vi "Main.vi"() -> ()   [LabVIEW 2014]
uses:
  Controls/FHandlerClusterTypedef.ctl
  Controls/FHandlerEnumTypedef.ctl
  Controls/CMWQCluster.ctl
  Controls/CMWQEnum.ctl
  Controls/CommentLogClusterTypedef.ctl
  Controls/CommentLogEnumTypedef.ctl
  <vilib>/Utility/sysdir.llb/System Directory Type.ctl
  Files/config/TableReference.ctl
  <vilib>/Utility/miscctls.llb/LVRowAndColumnTypeDef.ctl
  Controls/FGVisfileopen.ctl
  Controls/DataPack.ctl
  Controls/HeaderParameters.ctl
  Controls/MasterClusterTypedef.ctl
  Controls/MasterEnumTypedef.ctl
  Controls/ConfigFileWrite.ctl
  Controls/AddCommentParameters.ctl
panel:
  in  "PrintButton":bool
  out "Values going into graph":waveform(dbl)[](array[waveform])
  in  "Stop button":bool
  out "Error Out":errorcluster
  in  "Error In":errorcluster
  in  "Tab Control":T1(tab)
  out "Process GIF":bool
  in  "StartAcquisition":bool
  in  "StopAcq":bool
  in  "Clear-table":bool
  in  "Load Table from:":path=path "C:/LabVIEW Projects/coldex/COLDEX_LV_CG/trunk/Files/config/20150803_163022_configtable1.xlsx"
  in  "Table":i32(listbox)
  in  "LoadConfig":bool
  in  "ExportConfig":bool
  in  "File Path":path=path "C:/LabVIEW Projects/coldex/COLDEX_LV_CG/trunk/Documentation"
  in  "Comments:":string
  in  "Comment":bool
  in  "Clear Graph":bool
  out "Display Table":string[][](table)
  out "Output Waveforms":waveform(dbl)[](graph)
  # "EXPERIMENTAL DATA"
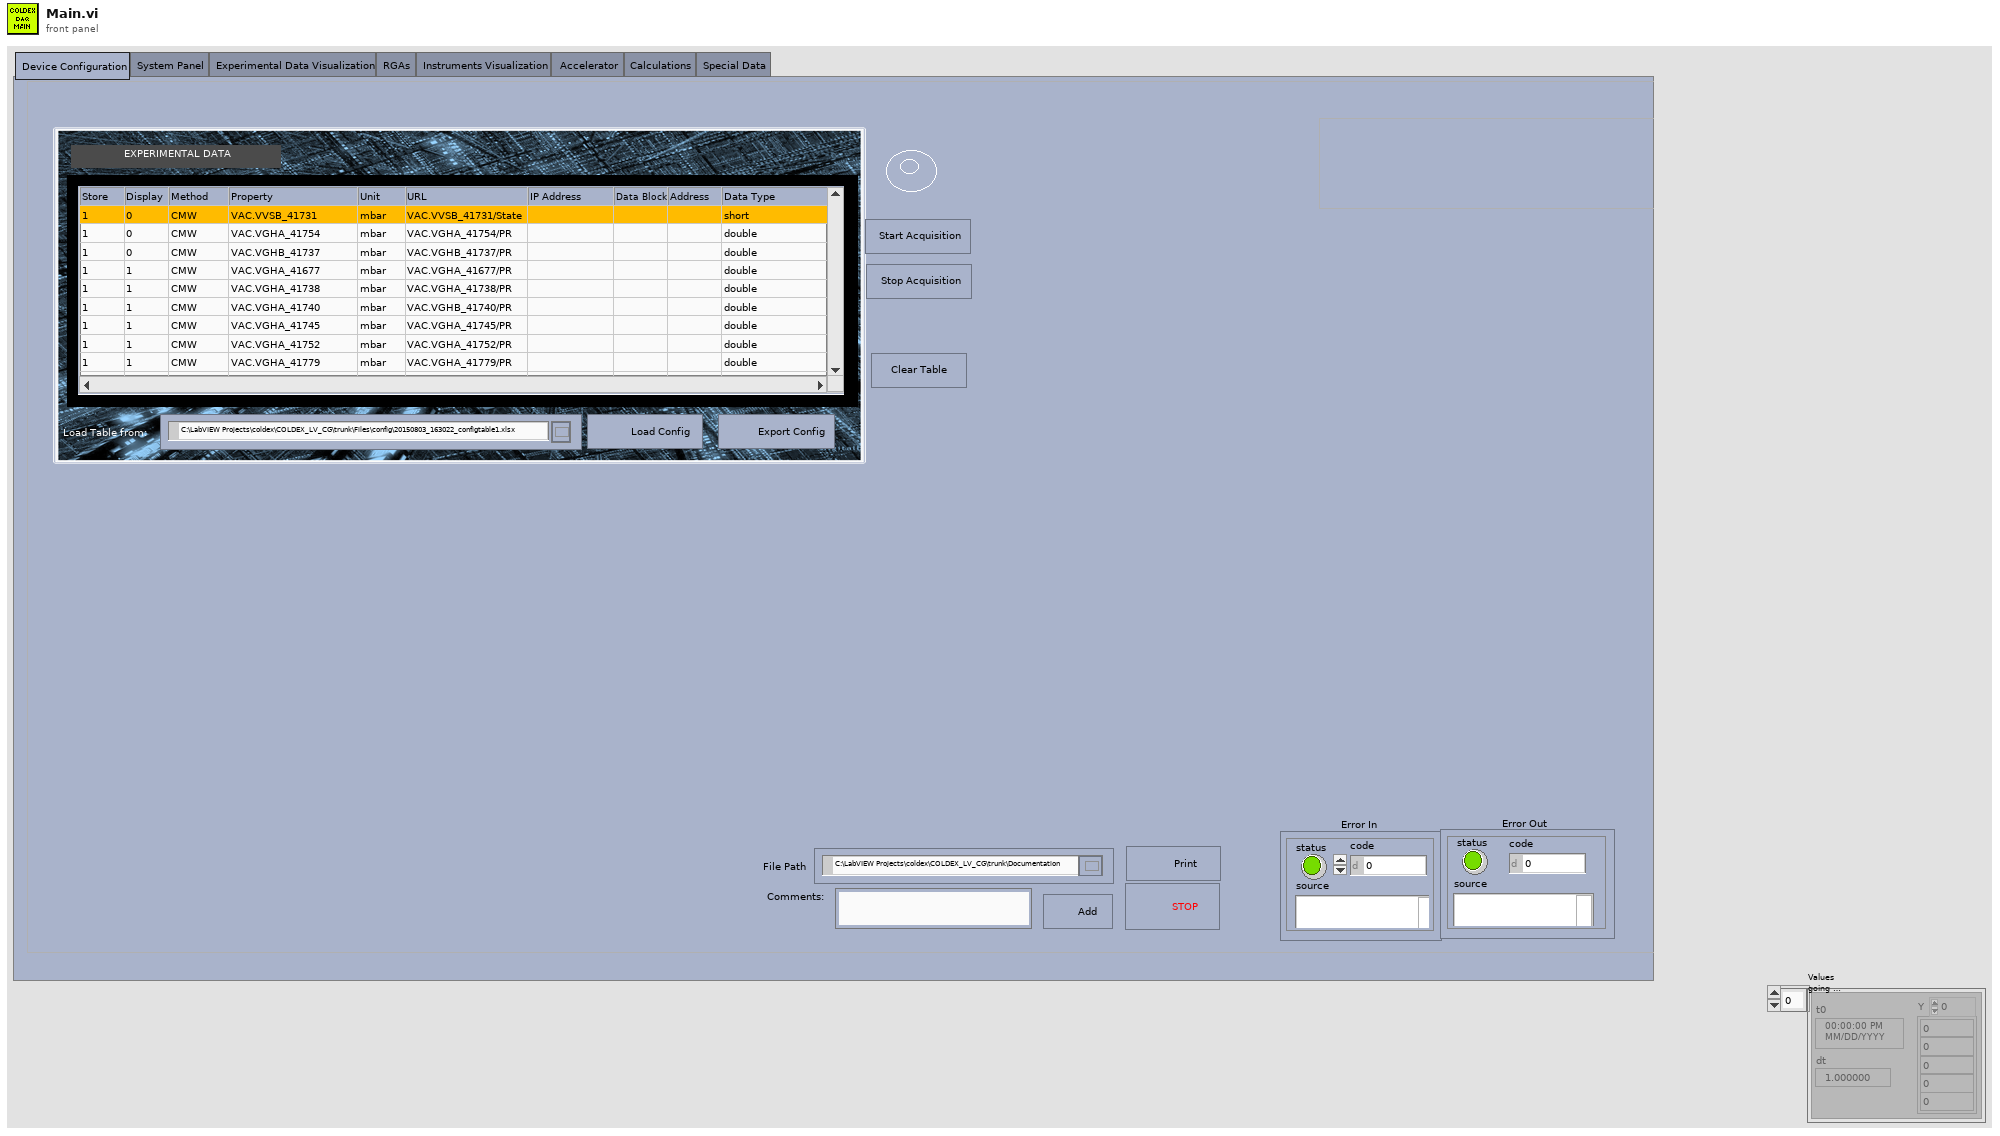
[diagram p1: front panel]
types:
  T1 = enum32{"Device Configuration", "System Panel", "Experimental Data Visualization", "RGAs", "Instruments Visualization", "Accelerator ", "Calculations", "Special Data"}
  T2 = typedef "FGVisfileopen.ctl" = enum16{"Read", "Write"}
  T3 = typedef "HeaderParameters.ctl" = cluster{"Property":string[], "Unit":string[], "Log Path":path}
  T4 = typedef "FHandlerClusterTypedef.ctl" = cluster{"File Variant":variant, "FileHandler Enum":T5}
  T5 = typedef "FHandlerEnumTypedef.ctl" = enum16{"InitLog", "CommentLog", "WriteExperimental", "WriteRGA", "WriteAccelerator", "WriteInstrument", "ClearLog", "ReadConfig", "WriteConfig", "ExitFH"}
  T6 = typedef "MasterClusterTypedef.ctl" = cluster{"DisplayVariant":variant, "DisplayEnum":T7}
  T7 = typedef "MasterEnumTypedef.ctl" = enum16{"Idle", "Initialize", "StartAcquisition", "StoreAcquisition", "PrintScreen", "AddComment", "ClearTable", "DisplayTable", "DisplayWaveforms", "ExportConfig", "LoadConfig", "Exit"}
  T8 = typedef "ConfigFileWrite.ctl" = cluster{"Headers":string[], "TableContent":string[][], "PathConfig":path}
  T9 = typedef "CommentLogClusterTypedef.ctl" = cluster{"variant":variant, "enum":T10}
  T10 = typedef "CommentLogEnumTypedef.ctl" = enum16{"AddComment", "Exit"}
  T11 = typedef "AddCommentParameters.ctl" = cluster{"PathConfig":path, "Comment":string}
  T12 = typedef "CMWQCluster.ctl" = cluster{"Variant":variant, "Enum":T13}
  T13 = typedef "CMWQEnum.ctl" = enum16{"Initialise", "Acquire", "Stop"}
  T14 = typedef "System Directory Type.ctl" = i32
  T15 = typedef "TableReference.ctl" = cluster{"Table Reference":refnum<vi>, "Cell Position":T16}
  T16 = typedef "LVRowAndColumnTypeDef.ctl" = cluster{"Row":i32, "Column":i32}
  T17 = typedef "LVPoint32TypeDef.ctl" = cluster{"Horizontal":i32, "Vertical":i32}
  T18 = cluster{"Start Row":i32, "Start Column":i32, "End Row":i32, "End Column":i32}
  T19 = typedef "DataPack.ctl" = cluster{"DataPack Array":cluster{"Method":string, "PropertyName":string, "Value":string, "Display?":string, "Unit":string}[], "current time":timestamp}
  T20 = cluster{"Method":string, "PropertyName":string, "Value":string, "Display?":string, "Unit":string}[]
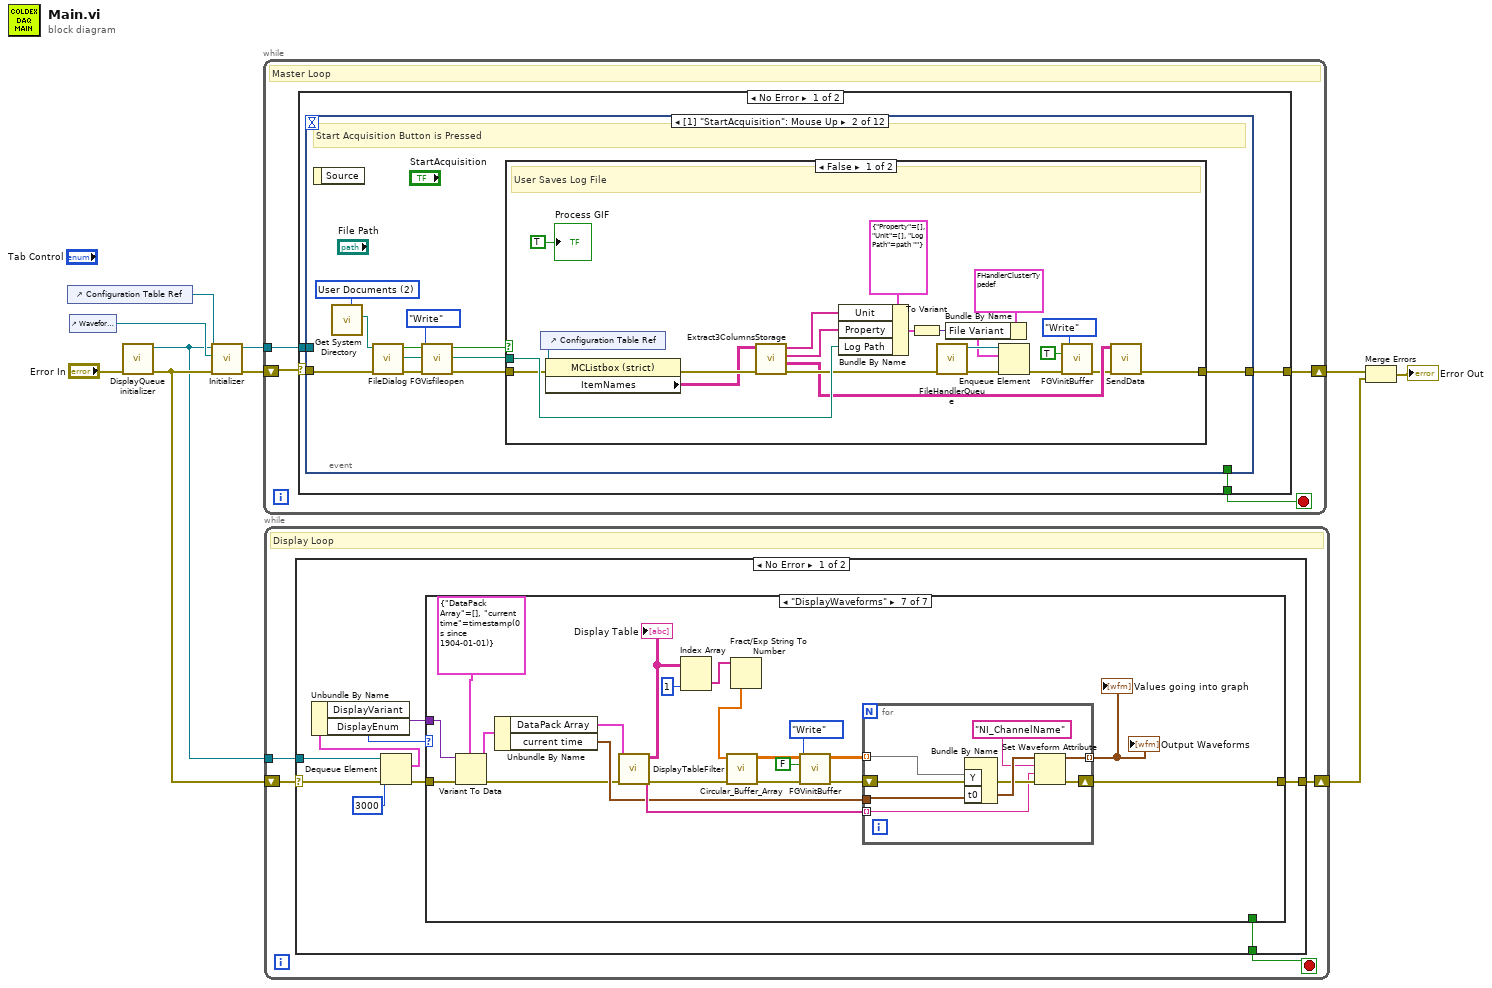
[diagram p0: block diagram]
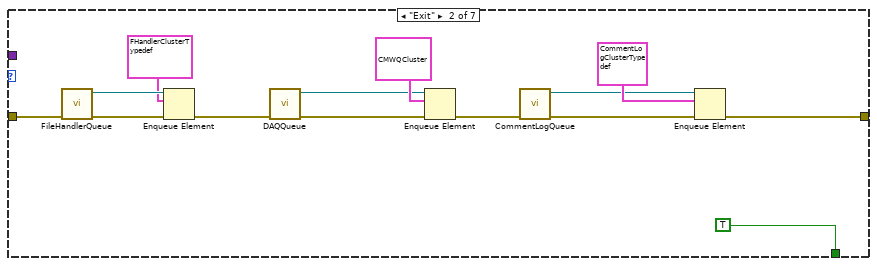
[diagram p3: hidden frame]
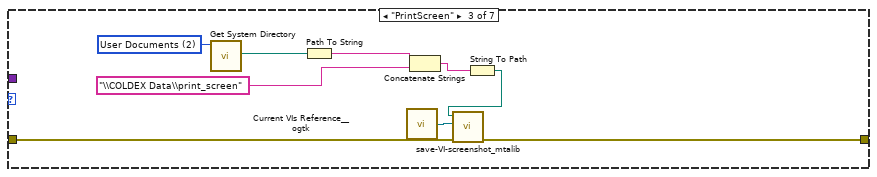
[diagram p4: hidden frame]
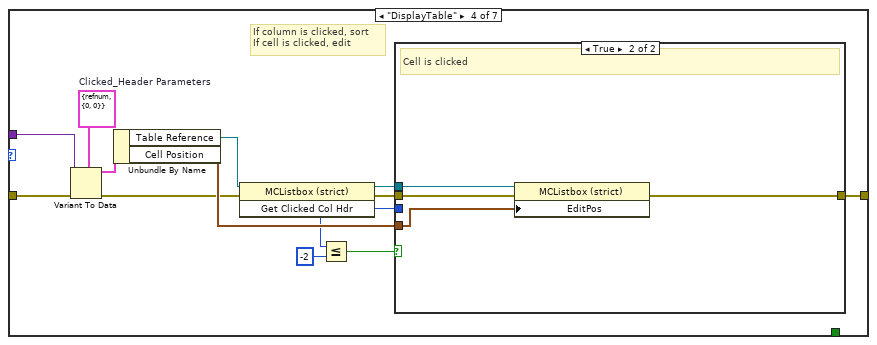
[diagram p5: hidden frame]
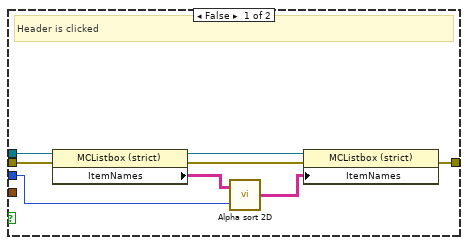
[diagram p6: hidden frame]
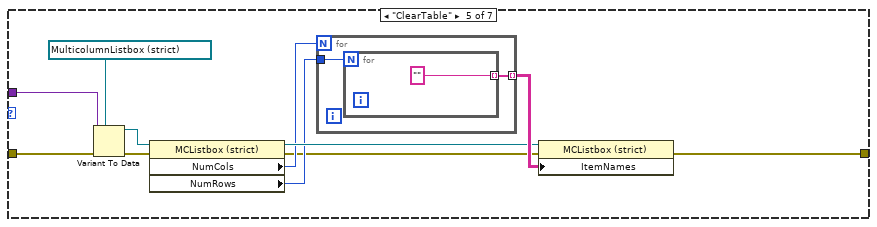
[diagram p7: hidden frame]
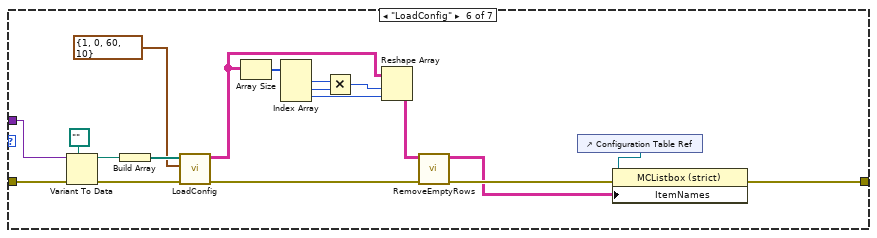
[diagram p8: hidden frame]
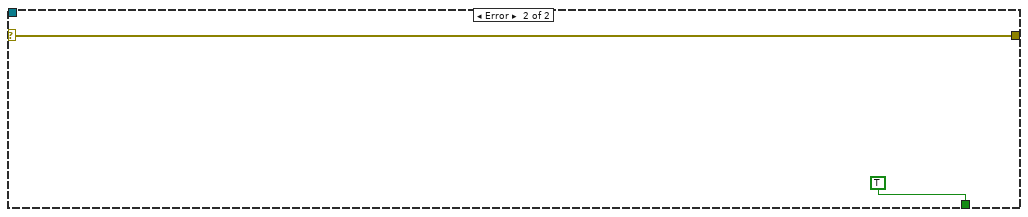
[diagram p9: hidden frame]
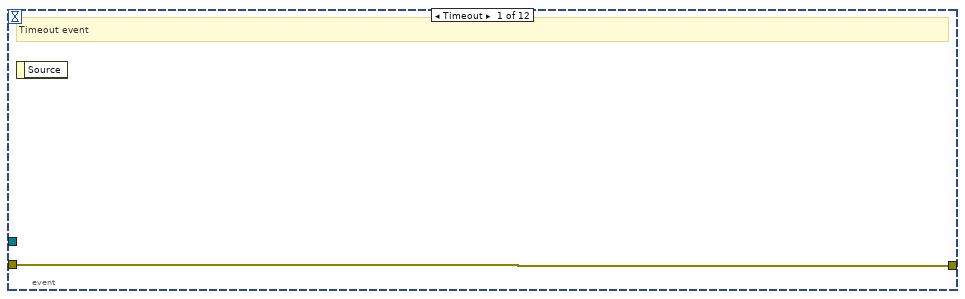
[diagram p10: hidden frame]
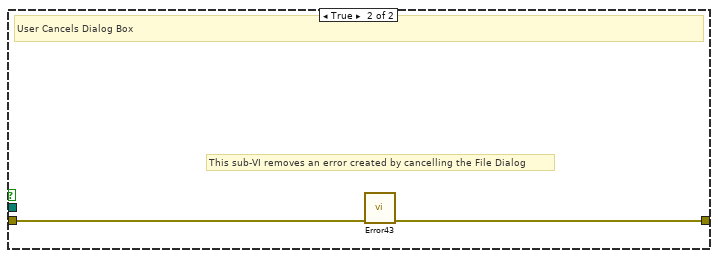
[diagram p11: hidden frame]
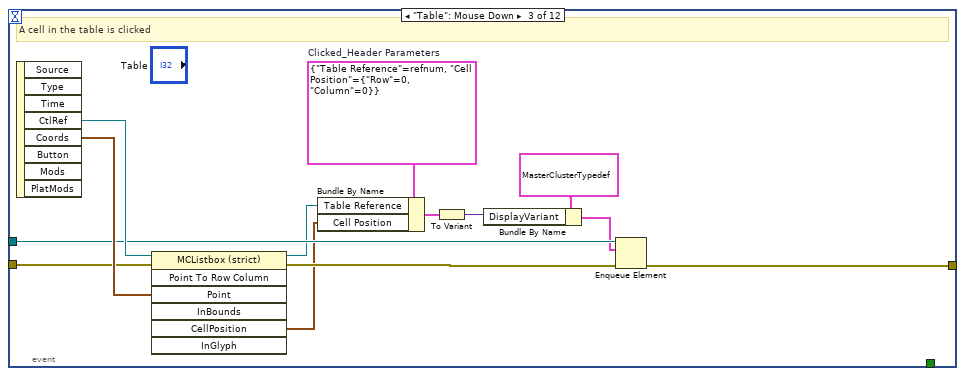
[diagram p12: hidden frame]
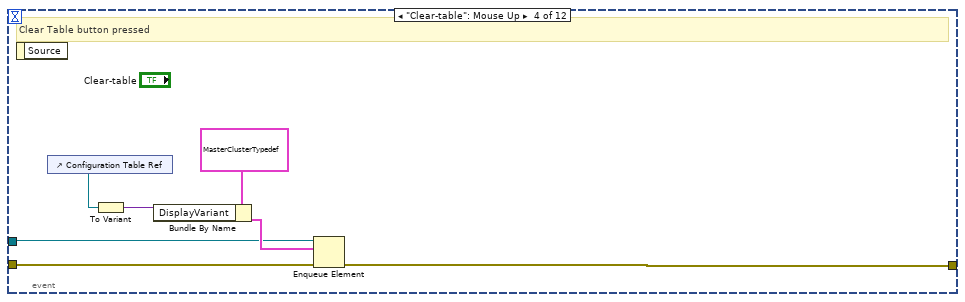
[diagram p13: hidden frame]
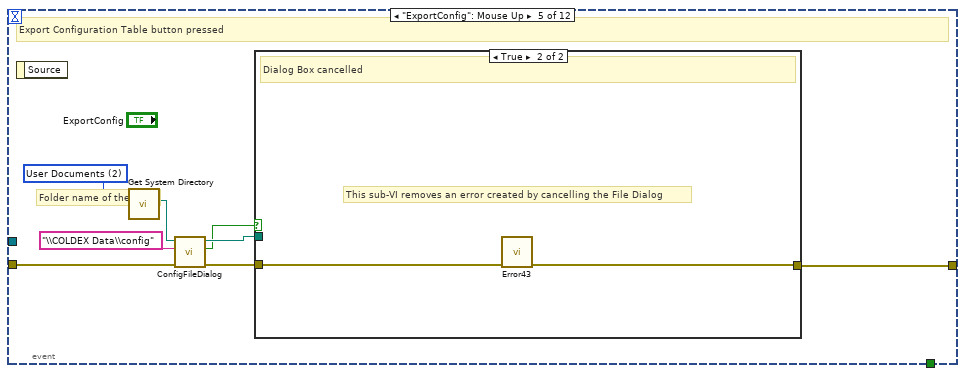
[diagram p14: hidden frame]
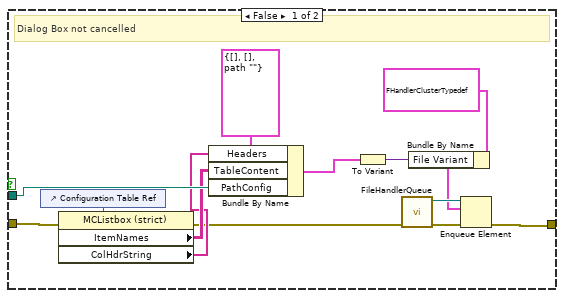
[diagram p15: hidden frame]
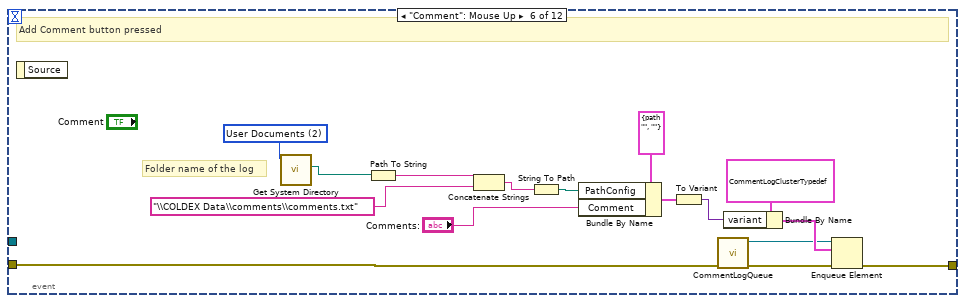
[diagram p16: hidden frame]
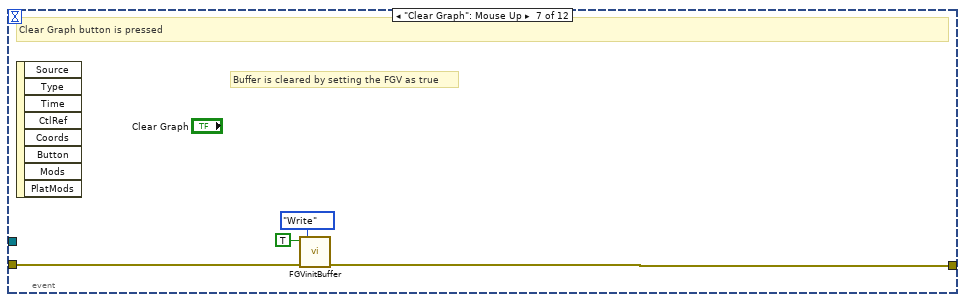
[diagram p17: hidden frame]
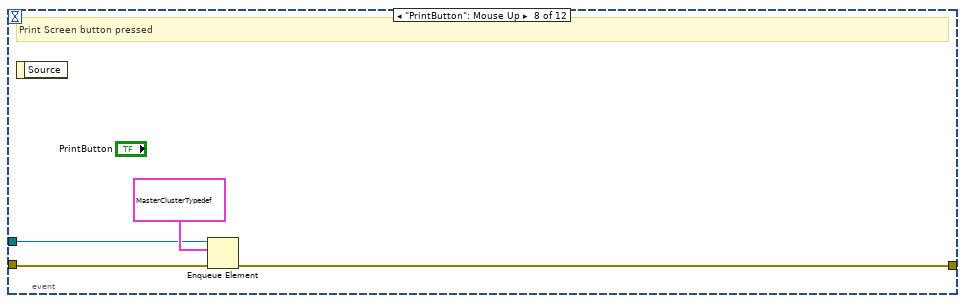
[diagram p18: hidden frame]
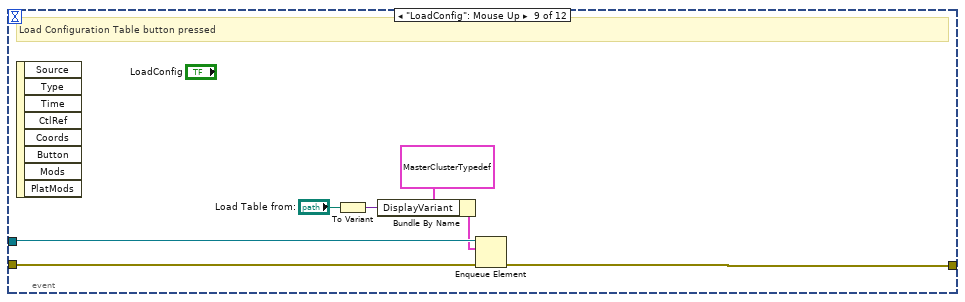
[diagram p19: hidden frame]
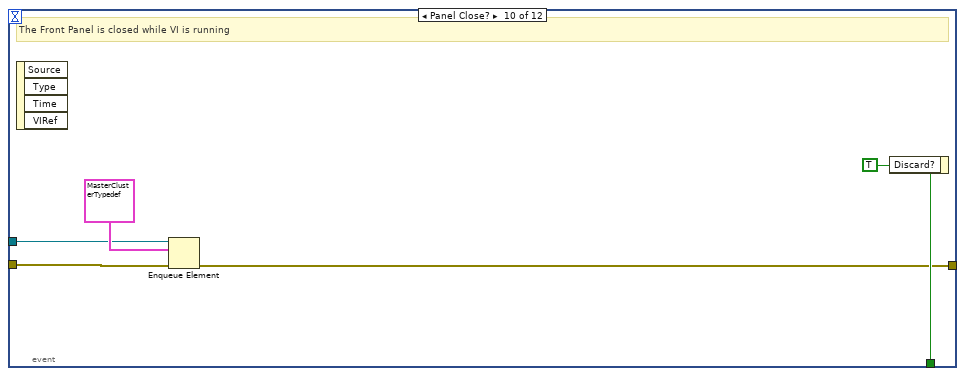
[diagram p20: hidden frame]
diagram:
  n1 = control-ref of="Configuration Table Ref"() -> (w5:refnum<vi>)
  n2 = control-ref of="Waveform Table Ref"() -> (w4:refnum<vi>)
  n3 = call "DisplayQueue initializer.vi"("error in"="Error In") -> ("error out"=w2:errorcluster, "queue out"=w1:refnum<queue>)  [unwired: 8 in]
  n4 = call "Initializer.vi"("Error In"=w2, "Display Table Ref"=w4, "Configuration Table Ref"=w5) -> ("Error Out"=w6:errorcluster)  [unwired: 8 in]
  n5 = while {
    tunnel: w1 -> [w10]
    shift-right: [w12] -> w7
    shift-left: w6 -> [w13]
    stop <- w11 stop-if-true
    # "Master Loop"
    n6 = case shown="No Error" w13 {
      selector: w13 -> [w16 w150]
      tunnel: [w15 w150] -> w12
      tunnel: [w14 TRUE] -> w11
      tunnel: w10 -> [w17 _]
      frame No Error {
        n7 = event shown="[1] \"StartAcquisition\": Mouse Up" {
          selector: _ -> [_ _ _ _ _ _ _ _ _ _ _ _]
          dyn-events: _ -> [_ _ _ _ _ _ _ _ _ _ _ _]
          timeout: _ -> [_ _ _ _ _ _ _ _ _ _ _ _]
          tunnel: w17 -> [_ _ w56 w67 _ _ _ w116 w124 w127 w138 _]
          tunnel: w16 -> [w18 w22 w62 w71 w79 w100 w114 w118 w126 w129 w133 w147]
          tunnel: [w18 w23 w61 w70 w76 w111 w113 w117 w125 w128 w137 w143] -> w15
          tunnel: [_ _ _ _ _ _ _ _ _ w131 TRUE _] -> w14
          event Timeout {
            # "Timeout event"
            n8 = event-data() -> ()  [unwired: 1 in, 1 out]
          }
          event "StartAcquisition": Mouse Up {
            w19 = T14 2 items=["User Home"=0, "User Desktop"=1, "User Documents"=2, "User Application Data"=3, "User Preferences"=4, "User Temporary"=5, "Public Documents"=6, "Public Application Data"=7, "Public Preferences"=8, "Public Cache"=13, "System Core Libraries"=9, "System Installed Libraries"=10, "Application Files"=11, "Boot Volume Root"=12] ("system directory type")
            # "Start Acquisition Button is Pressed"
            n9 = event-data() -> ()  [unwired: 1 in, 1 out]
            n10 = call <vilib>:"Get System Directory.vi"("system directory type"=w19) -> ("system directory"=w20:path)  [unwired: 10 in]
            n11 = call "FileDialog.vi"("Error In"=w22, "Path"=w20) -> ("Error Out"=w25:errorcluster, "cancelled dialog?"=w27:bool, "Output path"=w26:path)  [unwired: 7 in]
            n12 = call "FGVisfileopen.vi"("error in"=w25, "Read/Write?"=FGVisfileopen."Write" ("Write from FGV or Read from FGV?"), "Input Value"=w27) -> ("error out"=w21:errorcluster)  [unwired: 7 in, 1 out]
            n13 = case shown="False" w27 {
              tunnel: [w39 w51] -> w23
              tunnel: w26 -> [w40 _]
              tunnel: w21 -> [w33 w50]
              frame False {
                # "User Saves Log File"
                n14 = control-ref of="Configuration Table Ref"() -> (w43:refnum<vi>)
                n15 = property on="Property Node" class="MCListbox (strict)"(reference=w43, error in=w33) -> (error out=w49:errorcluster, "ItemNames"=w38:string[][])  [unwired: 1 out]
                n16 = call "Extract3ColumnsStorage.vi"("Error In"=w49, "Input Array"=w38) -> ("Error Out"=w36:errorcluster, "Filtered Array Out"=w32:string[][], "Property Out"=w35:string[], "Unit Out"=w34:string[])  [unwired: 6 in]
                n17 = Bundle By Name(cluster=T3 {"Property"=[], "Unit"=[], "Log Path"=path ""} ("Header Parameters"), "Unit"=w34, "Property"=w35, "Log Path"=w40) -> (w42:T3)
                n18 = To Variant(anything=w42) -> (Variant=w44:variant)
                n19 = call "FileHandlerQueue.vi"("error in"=w36) -> ("error out"=w48:errorcluster, "queue out"=w47:refnum<queue>)  [unwired: 8 in]
                n20 = Bundle By Name(cluster=T4 {"File Variant"=variant, "FileHandler Enum"=enum."InitLog"}, "File Variant"=w44) -> (w46:T4)
                n21 = Enqueue Element(queue=w47, element=w46, error in (no error)=w48) -> (error out=w31:errorcluster)  [unwired: 1 in, 2 out]
                n22 = call "FGVinitBuffer.vi"("error in"=w31, "Write/Read?"=FGVisfileopen."Write" ("Write from FGV or Read from FGV?"), "Input Value"=TRUE) -> ("error out"=w30:errorcluster)  [unwired: 7 in, 1 out]
                n23 = call "SendData.vi"("error in"=w30, "Input Array"=w32) -> ("error out"=w39:errorcluster)  [unwired: 9 in]
                "Process GIF" <- TRUE ("Process")
              }
              frame True {
                # "This sub-VI removes an error created by cancelling the File Dialog"
                # "User Cancels Dialog Box"
                n24 = call "Error43.vi"("error in"=w50) -> ("error out"=w51:errorcluster)  [unwired: 10 in]
              }
            }
          }
          event "Table": Mouse Down {
            w58 = T15 {"Table Reference"=refnum, "Cell Position"={"Row"=0, "Column"=0}}  # Clicked_Header Parameters
            # "A cell in the table is clicked"
            n25 = event-data() -> ("CtlRef"=w64:refnum<vi>, "Coords"=w63:T17)  [unwired: 1 in, 6 out]
            n26 = invoke class="MCListbox (strict)" method="Point To Row Column"(reference=w64, error in=w62, "Point"=w63) -> (reference out=w53:refnum<vi>, error out=w57:errorcluster, "CellPosition"=w52:T16)  [unwired: 4 in, 4 out]
            n27 = Bundle By Name(cluster=w58, "Table Reference"=w53, "Cell Position"=w52) -> (w59:T15)
            n28 = To Variant(anything=w59) -> (Variant=w55:variant)
            n29 = Bundle By Name(cluster=T6 {"DisplayVariant"=variant, "DisplayEnum"=enum."DisplayTable"}, "DisplayVariant"=w55) -> (w54:T6)
            n30 = Enqueue Element(queue=w56, element=w54, error in (no error)=w57) -> (error out=w61:errorcluster)  [unwired: 1 in, 2 out]
          }
          event "Clear-table": Mouse Up {
            # "Clear Table button pressed"
            n31 = event-data() -> ()  [unwired: 1 in, 1 out]
            n32 = control-ref of="Configuration Table Ref"() -> (w66:refnum<vi>)
            n33 = To Variant(anything=w66) -> (Variant=w69:variant)
            n34 = Bundle By Name(cluster=T6 {"DisplayVariant"=variant, "DisplayEnum"=enum."ClearTable"}, "DisplayVariant"=w69) -> (w68:T6)
            n35 = Enqueue Element(queue=w67, element=w68, error in (no error)=w71) -> (error out=w70:errorcluster)  [unwired: 1 in, 2 out]
          }
          event "ExportConfig": Mouse Up {
            w72 = T14 2 items=["User Home"=0, "User Desktop"=1, "User Documents"=2, "User Application Data"=3, "User Preferences"=4, "User Temporary"=5, "Public Documents"=6, "Public Application Data"=7, "Public Preferences"=8, "Public Cache"=13, "System Core Libraries"=9, "System Installed Libraries"=10, "Application Files"=11, "Boot Volume Root"=12] ("system directory type")
            # "Folder name of the log"
            # "Export Configuration Table button pressed"
            n36 = event-data() -> ()  [unwired: 1 in, 1 out]
            n37 = call <vilib>:"Get System Directory.vi"("system directory type"=w72) -> ("system directory"=w73:path)  [unwired: 10 in]
            n38 = call "ConfigFileDialog.vi"("Error In"=w79, "folder name"="\\COLDEX Data\\config" ("string"), "Path"=w73) -> ("Error Out"=w78:errorcluster, "cancelled dialog?"=w75:bool, "Output path"=w77:path)  [unwired: 6 in]
            n39 = case shown="True" w75 {
              tunnel: [w83 w94] -> w76
              tunnel: w77 -> [w87 _]
              tunnel: w78 -> [w81 w95]
              frame False {
                # "Dialog Box not cancelled"
                n40 = control-ref of="Configuration Table Ref"() -> (w89:refnum<vi>)
                n41 = property on="Property Node" class="MCListbox (strict)"(reference=w89, error in=w81) -> (error out=w80:errorcluster, "ItemNames"=w86:string[][], "ColHdrString"=w82:string[])  [unwired: 1 out]
                n42 = Bundle By Name(cluster=T8 {"Headers"=[], "TableContent"=[], "PathConfig"=path ""}, "Headers"=w82, "TableContent"=w86, "PathConfig"=w87) -> (w85:T8)
                n43 = To Variant(anything=w85) -> (Variant=w84:variant)
                n44 = call "FileHandlerQueue.vi"("error in"=w80) -> ("error out"=w93:errorcluster, "queue out"=w92:refnum<queue>)  [unwired: 8 in]
                n45 = Bundle By Name(cluster=T4 {"File Variant"=variant, "FileHandler Enum"=enum."WriteConfig"}, "File Variant"=w84) -> (w91:T4)
                n46 = Enqueue Element(queue=w92, element=w91, error in (no error)=w93) -> (error out=w83:errorcluster)  [unwired: 1 in, 2 out]
              }
              frame True {
                # "This sub-VI removes an error created by cancelling the File Dialog"
                # "Dialog Box cancelled"
                n47 = call "Error43.vi"("error in"=w95) -> ("error out"=w94:errorcluster)  [unwired: 10 in]
              }
            }
          }
          event "Comment": Mouse Up {
            w96 = T14 2 items=["User Home"=0, "User Desktop"=1, "User Documents"=2, "User Application Data"=3, "User Preferences"=4, "User Temporary"=5, "Public Documents"=6, "Public Application Data"=7, "Public Preferences"=8, "Public Cache"=13, "System Core Libraries"=9, "System Installed Libraries"=10, "Application Files"=11, "Boot Volume Root"=12] ("system directory type")
            # "Folder name of the log"
            # "Add Comment button pressed"
            n48 = event-data() -> ()  [unwired: 1 in, 1 out]
            n49 = call <vilib>:"Get System Directory.vi"("system directory type"=w96) -> ("system directory"=w97:path)  [unwired: 10 in]
            n50 = Path To String(path=w97) -> (string=w107:string)
            n51 = Concatenate Strings(w107, "\\COLDEX Data\\comments\\comments.txt" ("string")) -> (w108:string)
            n52 = String To Path(string=w108) -> (path=w105:path)
            n53 = Bundle By Name(cluster=T11 {"PathConfig"=path "", "Comment"=""}, "PathConfig"=w105, "Comment"="Comments:") -> (w102:T11)
            n54 = To Variant(anything=w102) -> (Variant=w110:variant)
            n55 = call "CommentLogQueue.vi"("error in"=w100) -> ("error out"=w99:errorcluster, "queue out"=w98:refnum<queue>)  [unwired: 8 in]
            n56 = Bundle By Name(cluster=T9 {"variant"=variant, "enum"=enum."AddComment"}, "variant"=w110) -> (w109:T9)
            n57 = Enqueue Element(queue=w98, element=w109, error in (no error)=w99) -> (error out=w111:errorcluster)  [unwired: 1 in, 2 out]
          }
          event "Clear Graph": Mouse Up {
            # "Buffer is cleared by setting the FGV as true"
            # "Clear Graph button is pressed"
            n58 = event-data() -> ()  [unwired: 1 in, 8 out]
            n59 = call "FGVinitBuffer.vi"("error in"=w114, "Write/Read?"=FGVisfileopen."Write" ("Write from FGV or Read from FGV?"), "Input Value"=TRUE) -> ("error out"=w113:errorcluster)  [unwired: 7 in, 1 out]
          }
          event "PrintButton": Mouse Up {
            # "Print Screen button pressed"
            n60 = event-data() -> ()  [unwired: 1 in, 1 out]
            n61 = Enqueue Element(queue=w116, element=T6 {"DisplayVariant"=variant, "DisplayEnum"=enum."PrintScreen"}, error in (no error)=w118) -> (error out=w117:errorcluster)  [unwired: 1 in, 2 out]
          }
          event "LoadConfig": Mouse Up {
            # "Load Configuration Table button pressed"
            n62 = event-data() -> ()  [unwired: 1 in, 8 out]
            n63 = To Variant(anything="Load Table from:") -> (Variant=w120:variant)
            n64 = Bundle By Name(cluster=T6 {"DisplayVariant"=variant, "DisplayEnum"=enum."LoadConfig"}, "DisplayVariant"=w120) -> (w121:T6)
            n65 = Enqueue Element(queue=w124, element=w121, error in (no error)=w126) -> (error out=w125:errorcluster)  [unwired: 1 in, 2 out]
          }
          event Panel Close? {
            w131 = TRUE ("Discard?")
            # "The Front Panel is closed while VI is running"
            n66 = event-data() -> ()  [unwired: 1 in, 4 out]
            n67 = Enqueue Element(queue=w127, element=T6 {"DisplayVariant"=variant, "DisplayEnum"=enum."Exit"}, error in (no error)=w129) -> (error out=w128:errorcluster)  [unwired: 1 in, 2 out]
            n68 = event-data("Discard?"=w131) -> ()  [unwired: 1 in, 1 out]
          }
          event "Stop button": Mouse Up {
            # "Stop button is pressed"
            n69 = event-data() -> ()  [unwired: 1 in, 1 out]
            n70 = property on="Process GIF" class="Bool (strict)"(error in=w133, "Value"=FALSE ("Process")) -> (error out=w132:errorcluster)  [unwired: 1 in, 1 out]
            n71 = Enqueue Element(queue=w138, element=T6 {"DisplayVariant"=variant, "DisplayEnum"=enum."Exit"}, error in (no error)=w132) -> (error out=w137:errorcluster)  [unwired: 1 in, 2 out]
          }
          event "StopAcq": Mouse Up {
            # "Stop Acquisition button is pressed"
            n72 = event-data() -> ()  [unwired: 1 in, 8 out]
            n73 = property on="Process GIF" class="Bool (strict)"(error in=w147, "Value"=FALSE ("Process")) -> (error out=w141:errorcluster)  [unwired: 1 in, 1 out]
            n74 = call "FGVstopacq.vi"("error in"=w141, "Write from FGV or Read from FGV?"=FGVisfileopen."Write", "Input Value"=TRUE) -> ("error out"=w140:errorcluster)  [unwired: 7 in, 1 out]
            n75 = call "DAQQueue.vi"("error in"=w140) -> ("error out"=w145:errorcluster, "queue out"=w144:refnum<queue>)  [unwired: 8 in]
            n76 = Enqueue Element(queue=w144, element=T12 {"Variant"=variant, "Enum"=enum."Stop"}, error in (no error)=w145) -> (error out=w143:errorcluster)  [unwired: 1 in, 2 out]
          }
        }
      }
      frame Error {
      }
    }
  }
  n77 = while {
    tunnel: w1 -> [w151]
    shift-right: [w153] -> w8
    shift-left: w2 -> [w154]
    stop <- w152 stop-if-true
    # "Display Loop"
    n78 = case shown="No Error" w154 {
      selector: w154 -> [w163 w275]
      tunnel: [w155 w275] -> w153
      tunnel: [w158 TRUE] -> w152
      tunnel: w151 -> [w161 _]
      frame No Error {
        n79 = Dequeue Element(queue=w161, timeout in ms (-1)=3000, error in (no error)=w163) -> (element=w159:T6, error out=w162:errorcluster)  [unwired: 2 out]
        n80 = Unbundle By Name(w159) -> ("DisplayVariant"=w156:variant, "DisplayEnum"=w157:T7)
        n81 = case shown="\"DisplayWaveforms\"" w157 {
          tunnel: [w164 w167 w185 w195 w213 w240 w251] -> w155
          tunnel: w162 -> [w164 w174 w186 w194 w222 w244 w265]
          tunnel: [_ TRUE _ _ _ _ _] -> w158
          tunnel: w156 -> [_ _ _ w200 w223 w243 w264]
          frame "Idle", Default {
          }
          frame "Exit" {
            n82 = call "FileHandlerQueue.vi"("error in"=w174) -> ("error out"=w177:errorcluster, "queue out"=w176:refnum<queue>)  [unwired: 8 in]
            n83 = Enqueue Element(queue=w176, element=T4 {"File Variant"=variant, "FileHandler Enum"=enum."ExitFH"}, error in (no error)=w177) -> (error out=w170:errorcluster)  [unwired: 1 in, 2 out]
            n84 = call "DAQQueue.vi"("error in"=w170) -> ("error out"=w172:errorcluster, "queue out"=w171:refnum<queue>)  [unwired: 8 in]
            n85 = Enqueue Element(queue=w171, element=T12 {"Variant"=variant, "Enum"=enum."Stop"}, error in (no error)=w172) -> (error out=w169:errorcluster)  [unwired: 1 in, 2 out]
            n86 = call "CommentLogQueue.vi"("error in"=w169) -> ("error out"=w168:errorcluster, "queue out"=w165:refnum<queue>)  [unwired: 8 in]
            n87 = Enqueue Element(queue=w165, element=T9 {"variant"=variant, "enum"=enum."Exit"}, error in (no error)=w168) -> (error out=w167:errorcluster)  [unwired: 1 in, 2 out]
          }
          frame "PrintScreen" {
            w179 = T14 2 items=["User Home"=0, "User Desktop"=1, "User Documents"=2, "User Application Data"=3, "User Preferences"=4, "User Temporary"=5, "Public Documents"=6, "Public Application Data"=7, "Public Preferences"=8, "Public Cache"=13, "System Core Libraries"=9, "System Installed Libraries"=10, "Application Files"=11, "Boot Volume Root"=12] ("system directory type")
            n88 = call <vilib>:"Get System Directory.vi"("system directory type"=w179) -> ("system directory"=w182:path)  [unwired: 10 in]
            n89 = Path To String(path=w182) -> (string=w183:string)
            n90 = call <userlib>:"Current VIs Reference__ogtk.vi"() -> ("Current VI's reference"=w187:refnum<vi>)  [unwired: 5 in]
            n91 = Concatenate Strings(w183, "\\COLDEX Data\\print_screen" ("string")) -> (w184:string)
            n92 = String To Path(string=w184) -> (path=w180:path)
            n93 = call <userlib>:"save-VI-screenshot_mtalib.vi"("error in (no error)"=w186, "Ctl Ref"=w187, "path to img"=w180) -> ("error out"=w185:errorcluster)  [unwired: 7 in, 1 out]
          }
          frame "DisplayTable" {
            w189 = T15 {"Table Reference"=refnum, "Cell Position"={"Row"=0, "Column"=0}}  # Clicked_Header Parameters
            # "If column is clicked, sort\nIf cell is clicked, edit"
            n94 = Variant To Data(error in=w194, type=w189, Variant=w200) -> (data=w199:T15, error out=w193:errorcluster)
            n95 = Unbundle By Name(w199) -> ("Table Reference"=w188:refnum<vi>, "Cell Position"=w196:T16)
            n96 = invoke class="MCListbox (strict)" method="Get Clicked Col Hdr"(reference=w188, error in=w193) -> (reference out=w197:refnum<vi>, error out=w198:errorcluster, "Get Clicked Column Header"=w190:i32)  [unwired: 1 in]
            n97 = Less Or Equal?(x=w190, y=-2) -> (x <= y?=w192:bool)
            n98 = case shown="True" w192 {
              tunnel: w198 -> [w207 w212]
              tunnel: w197 -> [w208 w211]
              tunnel: w196 -> [_ w210]
              tunnel: w190 -> [w203 _]
              tunnel: [w204 w209] -> w195
              frame False {
                # "Header is clicked"
                n99 = property on="Property Node" class="MCListbox (strict)"(reference=w208, error in=w207) -> (reference out=w206:refnum<vi>, error out=w205:errorcluster, "ItemNames"=w202:string[][])
                n100 = call "Alpha sort 2D.vi"("Column Number"=w203, "Input Array"=w202) -> ("Sorted Array"=w201:string[][])
                n101 = property on="Property Node" class="MCListbox (strict)"(reference=w206, error in=w205, "ItemNames"=w201) -> (error out=w204:errorcluster)  [unwired: 1 out]
              }
              frame True {
                # "Cell is clicked"
                n102 = property on="Property Node" class="MCListbox (strict)"(reference=w211, error in=w212, "EditPos"=w210) -> (error out=w209:errorcluster)  [unwired: 1 out]
              }
            }
          }
          frame "ClearTable" {
            n103 = Variant To Data(error in=w222, type=refnum<vi> refnum ("Table"), Variant=w223) -> (data=w219:refnum<vi>, error out=w215:errorcluster)
            n104 = property on="Property Node" class="MCListbox (strict)"(reference=w219, error in=w215) -> (reference out=w218:refnum<vi>, error out=w214:errorcluster, "NumCols"=w217:u32, "NumRows"=w216:u32)
            n105 = for {
              N: w217 -> [_]
              tunnel: [w225] -> w220 mode=indexing
              tunnel: w216 -> [w224]
              n106 = for {
                N: w224 -> [_]
                tunnel: [""] -> w225 mode=indexing
              }
            }
            n107 = property on="Property Node" class="MCListbox (strict)"(reference=w218, error in=w214, "ItemNames"=w220) -> (error out=w213:errorcluster)  [unwired: 1 out]
          }
          frame "LoadConfig" {
            n108 = Variant To Data(error in=w244, type=path "" ("Load Table from:"), Variant=w243) -> (data=w242:path, error out=w232:errorcluster)
            n109 = Build Array(w242) -> (w234:path[])
            n110 = call "LoadConfig.vi"("error in (no error)"=w232, "Start and End"=T18 {"Start Row"=1, "Start Column"=0, "End Row"=60, "End Column"=10}, "Array"=w234) -> ("error out"=w230:errorcluster, "data"=w231:string[][][])  [unwired: 5 in]
            n111 = Array Size(array=w231) -> (size(s)=w239:i32[])
            n112 = Index Array(array=w239) -> (element #1=w237:i32, element #2=w238:i32, element #3=w235:i32)  [unwired: 3 in]
            n113 = Multiply(x=w237, y=w238) -> (x*y=w236:i32)
            n114 = Reshape Array(w231, w236, w235) -> (w227:string[][])
            n115 = call "RemoveEmptyRows.vi"("Error In"=w230, "Input array with empty rows"=w227) -> ("Error Out"=w229:errorcluster, "array w/ subset deleted"=w228:string[][])  [unwired: 8 in]
            n116 = control-ref of="Configuration Table Ref"() -> (w241:refnum<vi>)
            n117 = property on="Property Node" class="MCListbox (strict)"(reference=w241, error in=w229, "ItemNames"=w228) -> (error out=w240:errorcluster)  [unwired: 1 out]
          }
          frame "DisplayWaveforms" {
            n118 = Variant To Data(error in=w265, type=T19 {"DataPack Array"=[], "current time"=timestamp(0 s since 1904-01-01)}, Variant=w264) -> (data=w263:T19, error out=w255:errorcluster)
            n119 = Unbundle By Name(w263) -> ("DataPack Array"=w254:T20, "current time"=w256:timestamp)
            n120 = call "DisplayTableFilter.vi"("Error In"=w255, "DataPack Array"=w254) -> ("Error out"=w246:errorcluster, "Propertynames"=w257:string[], "Table Array"=w262:string[][])  [unwired: 7 in]
            "Display Table" <- w262
            n121 = Index Array(array=w262, index (col)=1 ("disabled index (col)")) -> (element=w260:string[])  [unwired: 1 in]
            n122 = Fract/Exp String To Number(string=w260) -> (number=w247:dbl[])  [unwired: 3 in, 1 out]
            n123 = call "Circular_Buffer_Array.vi"("Error In"=w246, "Array"=w247) -> ("Error Out"=w250:errorcluster, "output array"=w259:dbl[][])  [unwired: 8 in]
            n124 = call "FGVinitBuffer.vi"("error in"=w250, "Write/Read?"=FGVisfileopen."Write" ("Write from FGV or Read from FGV?"), "Input Value"=FALSE) -> ("error out"=w249:errorcluster)  [unwired: 7 in, 1 out]
            n125 = for {
              tunnel: w259 -> [w268] mode=indexing
              tunnel: w256 -> [w266]
              tunnel: [w272] -> w258 mode=indexing
              tunnel: w257 -> [w267] mode=indexing
              shift-right: [w271] -> w251
              shift-left: w249 -> [w270]
              n126 = Bundle By Name("Y"=w268, "t0"=w266) -> (w273:waveform(dbl))  [unwired: 1 in]
              n127 = Set Waveform Attribute(4:w270, 5:w267, 6:"NI_ChannelName" ("Channel Name"), 7:w273) -> (0:w271:errorcluster, 3:w272:waveform(dbl))  [unwired: 1 out]
            }
            "Output Waveforms" <- w258
            "Values going into graph" <- w258
          }
        }
      }
      frame Error {
      }
    }
  }
  n128 = Merge Errors(w7, w8) -> (→"Error Out":errorcluster)
